vi "Ping.vi"(10 "hostNameOrAddress":string="192.168.127.2", 11 "secIn":i32) -> (1 "Status":i32(ring) items=["Success"=0, "DestinationNetworkUnreachable"=11002, "DestinationHostUnreachable"=11003, "DestinationProhibited, DestinationProtocolUnreachable"=11004, "DestinationPortUnreachable"=11005, "NoResources"=11006, "BadOption"=11007, "HardwareError"=11008, "PacketTooBig"=11009, "TimedOut"=11010, "BadRoute"=11012, "TtlExpired"=11013, "TtlReassemblyTimeExceeded"=11014, "ParameterProblem"=11015, "SourceQuench"=11016, "BadDestination"=11018, "DestinationUnreachable"=11040, "TimeExceeded"=11041, "BadHeader"=11042, "UnrecognizedNextHeader"=11043, "IcmpError"=11044, "DestinationScopeMismatch"=11045, "Unknown"=-1], 2 "bolStatus":bool, 3 "secOut":i32)   [LabVIEW 2017]
panel:
  in  "hostNameOrAddress 2":string="192.168.127.2"
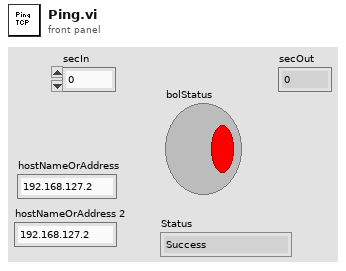
[diagram p1: front panel]
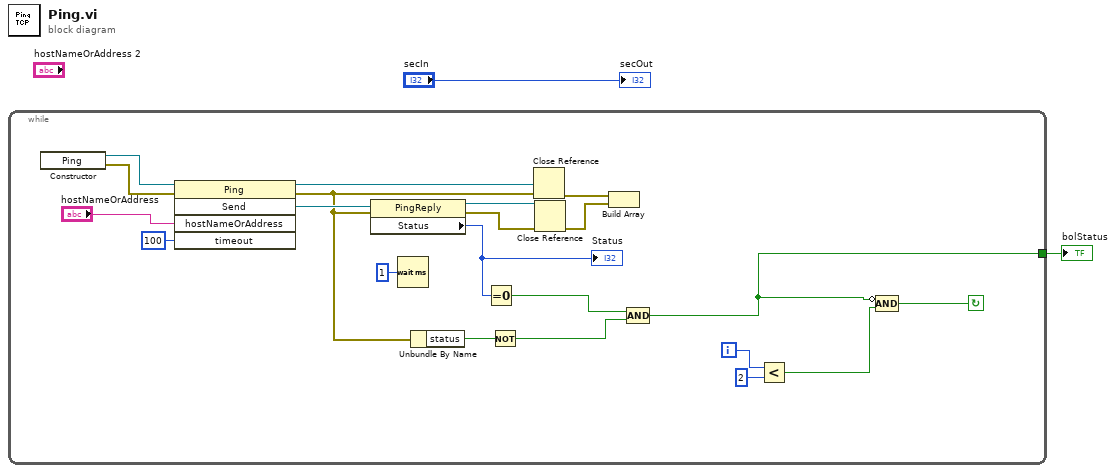
[diagram p0: block diagram]
diagram:
  n1 = while {
    tunnel: [w3] -> w1
    i -> [w12]
    stop <- w13 continue-if-true
    n2 = constructor class="Ping"() -> (reference out=w21:refnum<k24>, error out=w9:errorcluster)  [unwired: 3 in, 1 out]
    n3 = invoke class="Ping" method="Send"(reference=w21, error in=w9, "hostNameOrAddress"="hostNameOrAddress", "timeout"=100) -> (reference out=w23:refnum<k24>, error out=w6:errorcluster, "Send"=w20:refnum<k24>)  [unwired: 1 in, 2 out]
    n4 = property class="PingReply"(reference=w20, error in=w6) -> (reference out=w22:refnum<k24>, error out=w8:errorcluster, "Status"=w17:i32)
    "Status" <- w17
    n5 = Wait (ms)(milliseconds to wait=u32 1) -> ()  [unwired: 1 out]
    n6 = Unbundle By Name(w6) -> ("status"=w5:bool)
    n7 = Equal To 0?(x=w17) -> (x = 0?=w7:bool)
    n8 = Not(x=w5) -> (.not. x?=w4:bool)
    n9 = Close Reference(reference=w23, error in (no error)=w6) -> (error out=w11:errorcluster)
    n10 = Close Reference(reference=w22, error in (no error)=w8) -> (error out=w10:errorcluster)
    n11 = Build Array(w11, w10) -> ()  [unwired: 1 out]
    n12 = Compound Arithmetic op=AND(w7, w4) -> (w3:bool)
    n13 = Less?(x=w12, y=2) -> (x < y?=w15:bool)
    n14 = Compound Arithmetic op=AND(invert w3, w15) -> (w13:bool)
  }
  "bolStatus" <- w1
  "secOut" <- "secIn"
